vi "Test Read.vi"(6 "Append Index":i32, 8 "error in (no error)":errorcluster, 10 "command":string="SELECT * FROM test_table where my_dbl>0.99;", 11 "Data.PG in":refnum<class "Data.PG.lvclass">) -> (0 "error out":errorcluster, 1 "Notes":string, 2 "Data (Dictionary)":T1[](array[typedef]), 3 "Data.PG out":refnum<class "Data.PG.lvclass">, 4 "Result":string[][](array[string]), 5 "Path out":path)   [LabVIEW 2020, in "Data.PG.lvclass"]
uses:
  Data.PG.lvclass
  C:/Users/Phil/levylab/LV-to-ITX/src/Data/Data.lvclass
  Data/Typedefs/Dictionary--cluster.ctl
  <vilib>/JDP Science/PostgreSQL Library/Connection/PQ Connection.lvclass
  Data.PG.lvclass/Data.PG.ctl
  Data/Typedefs/Operation--enum.ctl
  Data/Data.lvclass/Data.ctl
  <vilib>/JDP Science/PostgreSQL Library/Result/PQ Result.lvclass/PQ Result.ctl
  <vilib>/JDP Science/PostgreSQL Library/Connection/Execute Command (2D string results).vi
  <vilib>/JDP Science/PostgreSQL Library/Result/Clear.vi
  <vilib>/JDP Science/PostgreSQL Library/Connection/Execute Command (Result).vi
  <vilib>/JDP Science/PostgreSQL Library/Connection/Execute (Return first result with rows).vi
  <vilib>/JDP Science/PostgreSQL Library/Connection/Single Command with parameters.vi
  <vilib>/JDP Science/PostgreSQL Library/Result/Get all results as 2D strings array.vi
  Data/Data.lvclass
  <vilib>/JDP Science/PostgreSQL Library/Result/PQ Result.lvclass
panel:
  out "size(s)":i32[](array[numeric])
  # "MNK"
  # "fsfdfsglkjjjb"
  # "SAMPLE"
  # "GUID EXPT#?"
  # "time"
  # "INST"
  # "ID#"
  # "Vsg"
  # "T"
  # "B"
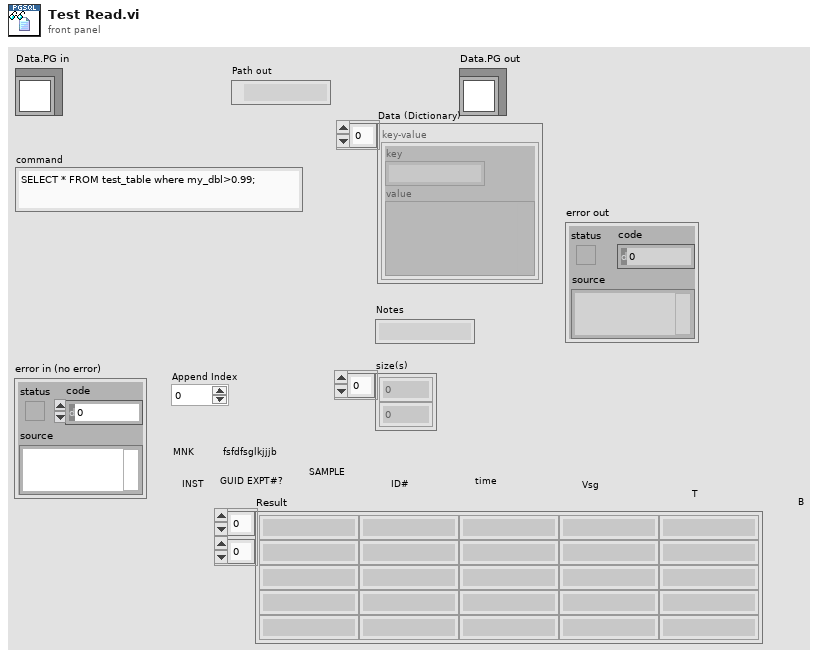
[diagram p1: front panel]
types:
  T1 = typedef "Data.lvclass/Dictionary--cluster.ctl" = cluster{"key":string, "value":variant}
  T2 = typedef "Data.lvclass/Operation--enum.ctl" = enum16{"Read", "Write", "Write + Append"}
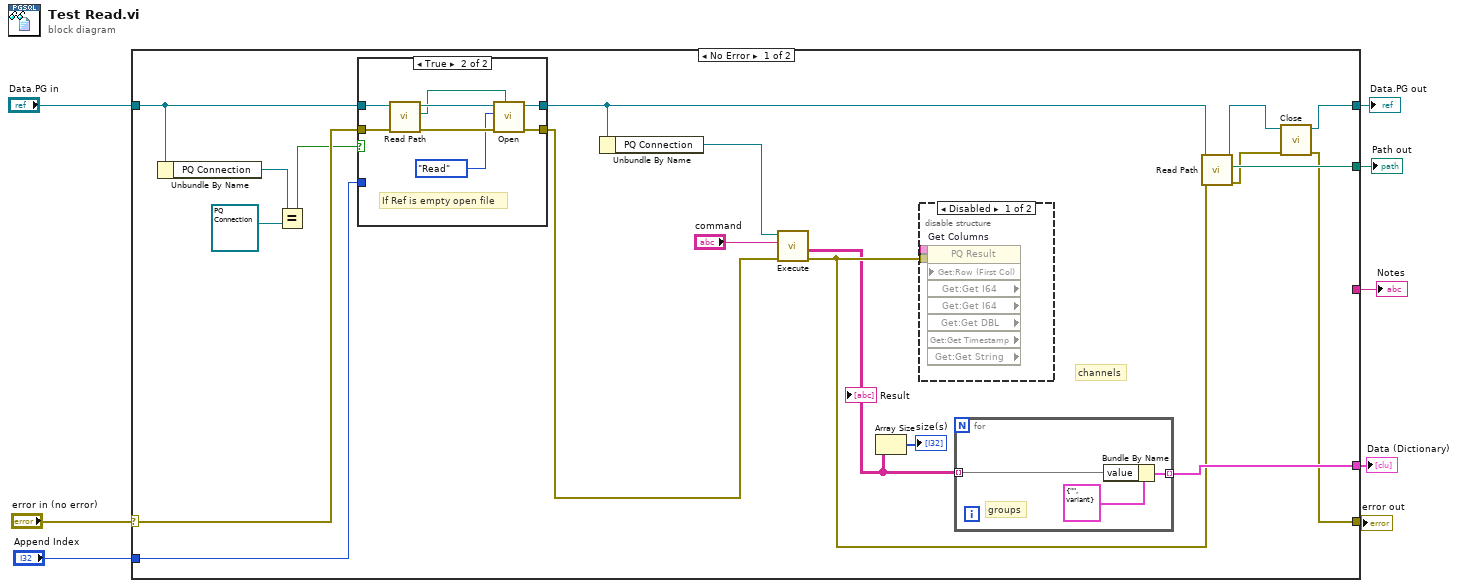
[diagram p0: block diagram]
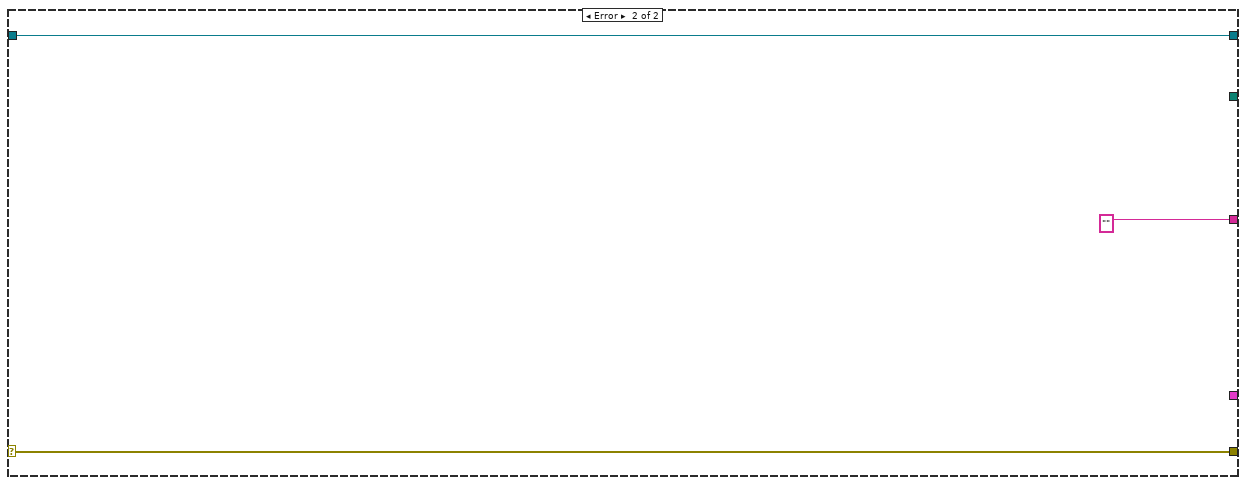
[diagram p4: hidden frame]
diagram:
  n1 = case shown="No Error" "error in (no error)" {
    selector: "error in (no error)" -> [w24 w45]
    tunnel: "Data.PG in" -> [w25 w44]
    tunnel: [w11 w44] -> w7
    tunnel: [w9 w45] -> w6
    tunnel: [w26 _] -> w5
    tunnel: "Append Index" -> [w20 _]
    tunnel: [w27 _] -> w1
    tunnel: [_ ""] -> w2
    frame No Error {
      # "channels"
      n2 = Unbundle By Name(w25) -> ("PQ Connection"=w22:refnum<class "PQ Connection.lvclass">)
      n3 = Equal?(x=w22, y=refnum<class "PQ Connection.lvclass"> refnum ("PQ Connection")) -> (x = y?=w21:bool)
      n4 = case shown="True" w21 {
        tunnel: w25 -> [w33 w41]
        tunnel: [w33 w42] -> w19
        tunnel: [w34 w38] -> w18
        tunnel: w24 -> [w34 w37]
        tunnel: w20 -> [_ _]
        frame False {
        }
        frame True {
          # "If Ref is empty open file"
          n5 = call "Read Path.vi"("error in (no error)"=w37, "Data Save"=w41) -> ("error out"=w40:errorcluster, "Path"=w36:path, "Data Save out"=w39:refnum<class "Data.PG.lvclass">)  [unwired: 7 in]
          n6 = call-dynamic "Open.vi"("Path"=w36, "error in (no error)"=w40, "Operation"=Operation--enum."Read", "Data.PG in"=w39) -> ("error out"=w38:errorcluster, "Data.PG out"=w42:refnum<class "Data.PG.lvclass">)  [unwired: 6 in]
        }
      }
      n7 = Unbundle By Name(w19) -> ("PQ Connection"=w16:refnum<class "PQ Connection.lvclass">)
      n8 = call-poly <vilib>:"Execute.vi"("error in (no error)"=w18, "SQL"="command", "PQ Connection in"=w16) -> ("error out"=w15:errorcluster, "Result"=w14:string[][])  [unwired: 5 in, 2 out]
      "Result" <- w14
      n9 = Array Size(array=w14) -> (size(s)=→"size(s)":i32[])
      n10 = disable-structure shown="Disabled" {
        disable-tunnel: _ -> [w32 _]
        disable-tunnel: w15 -> [w31 _]
        frame Disabled {
          n11 = property on="Get Columns" class="PQ Result" props=["Get:Row (First Col)", "Get:Get I64", "Get:Get I64", "Get:Get DBL", "Get:Get Timestamp", "Get:Get String"](reference=w32, error in=w31) -> ()  [unwired: 1 in, 7 out]
        }
        frame Enabled {
        }
      }
      n12 = for {
        tunnel: [w30] -> w27 mode=indexing
        tunnel: w14 -> [w28] mode=indexing
        # "groups"
        n13 = Bundle By Name(cluster=T1 {"key"="", "value"=variant} ("key-value"), "value"=w28) -> (w30:T1)
      }
      n14 = call "Read Path.vi"("error in (no error)"=w15, "Data Save"=w19) -> ("error out"=w10:errorcluster, "Path"=w26:path, "Data Save out"=w12:refnum<class "Data.PG.lvclass">)  [unwired: 7 in]
      n15 = call-dynamic "Close.vi"("error in (no error)"=w10, "Data.PG in"=w12) -> ("error out"=w9:errorcluster, "Data.PG out"=w11:refnum<class "Data.PG.lvclass">)  [unwired: 8 in]
    }
    frame Error {
    }
  }
  "error out" <- w6
  "Data.PG out" <- w7
  "Path out" <- w5
  "Data (Dictionary)" <- w1
  "Notes" <- w2
